vi "AppendSingle.vi"(6 "Only append if new?":bool=TRUE caption="Only append if new? (T)", 8 "Error to append":errorcluster, 9 "Error in":errorcluster) -> (1 "Appended errors out":errorcluster)   [LabVIEW 2017, in "GPError.lvlib"]
doc: "Appends <B>Error to append</B> to <B>Error in</B>.\n\nAppending errors preserves the contents of the two error clusters opposed to merging errors (with the built-in 'Merge Errors' function) which only keeps the highest priority error and scraps the rest. Appending errors maintains all error information inside the Source string of a single error cluster. Built-in, overridden and custom errors are supported.\n\nUse the SplitAppended function to split an appended error cluster into an array of individual error clusters.\n\nOnly errors and warnings are appended, any 'No error' is skipped.\n\nThe optional <B>Only append if new?</B> will, if set to True (which is the default setting), make this VI test if <B>Error to append</B> is already present in <B>Error in</B>. If that is the case (possibly as an earlier appended error) then no new append will occur. This feature is valuable if you append errors in a loop and risk encountering the same error over and over again, but you don't want to keep piling up all new copies of the same error. Set <B>Only append if new?</B> to False to append unconditionally.\n\nThis function considers two errors equal only if their code, status, source and description fields are all identical. Two errors that differ only in timestamp are considered equal as well however, the one already present in <B>Error in</B> staying put.\n\nThis VI might change the order of the appended errors, as it will always seek to move at least one error in front of any warnings in the appended error collection. This is to avoid any of the built-in LabVIEW functions wrongfully overwriting an appended error with its own error, which it will if a warning is the top-most value in the appended error collection.\n\nThis VI is reentrant.\n\nSteen Schmidt\nGPower\n18/7 2013"
uses:
  GPError.lvlib
  <vilib>/Utility/error.llb/DialogType.ctl
panel:
  # "Copyright © 2013\nSteen Schmidt, GPower\nSee enclosed license file for terms and conditions"
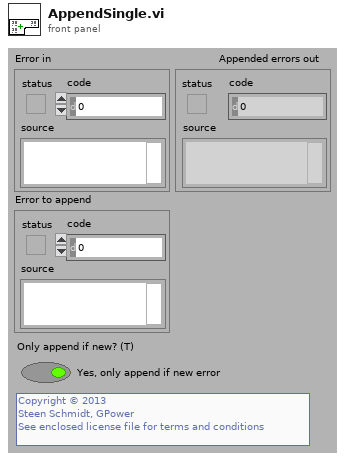
[diagram p1: front panel]
types:
  T1 = typedef "DialogType.ctl" = u16
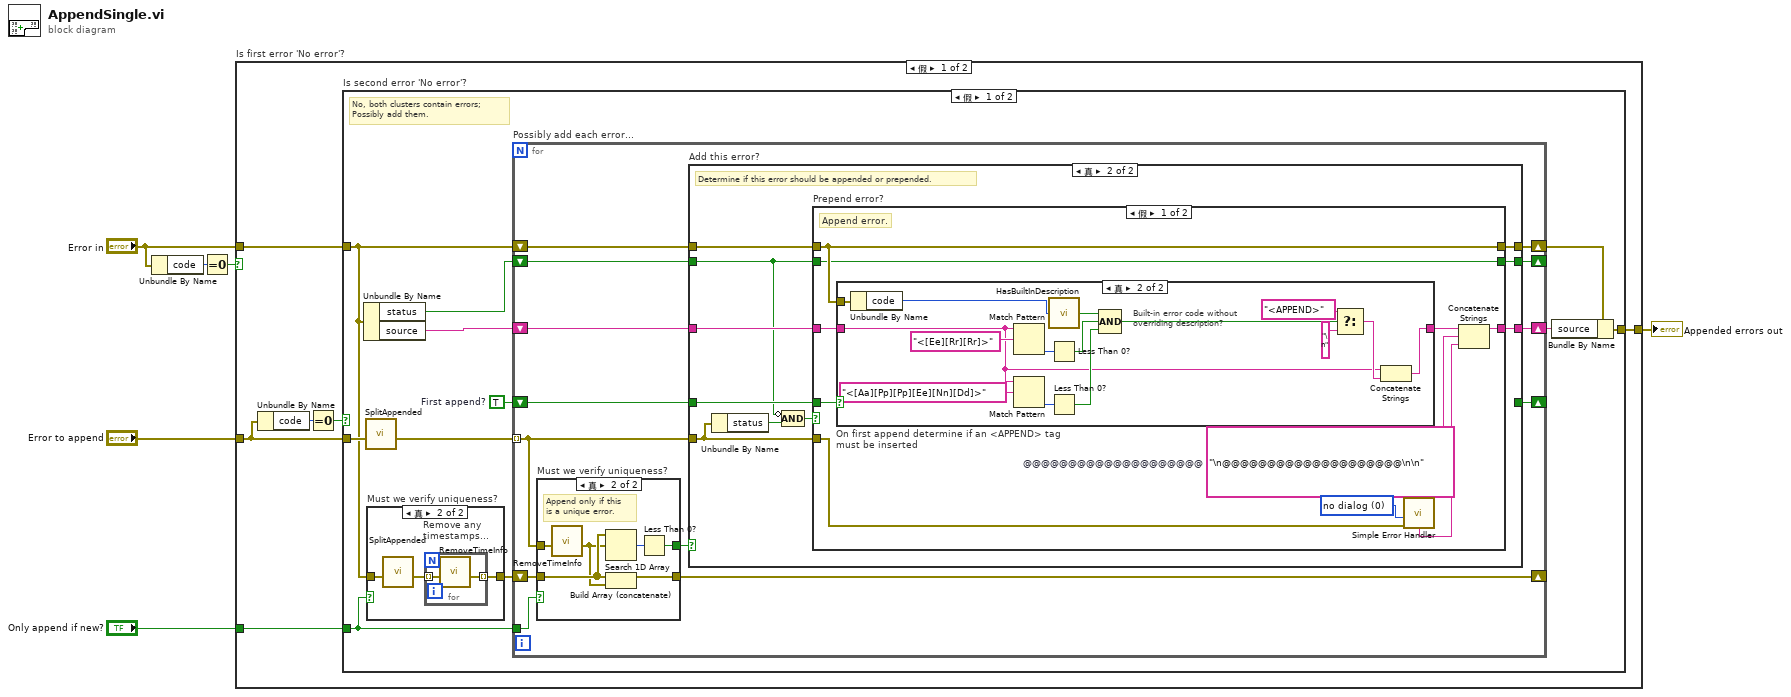
[diagram p0: block diagram]
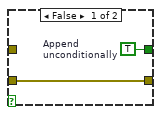
[diagram p3: hidden frame]
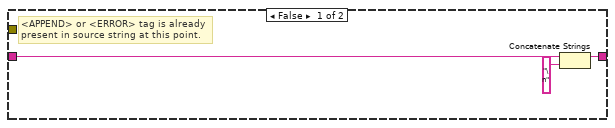
[diagram p5: hidden frame]
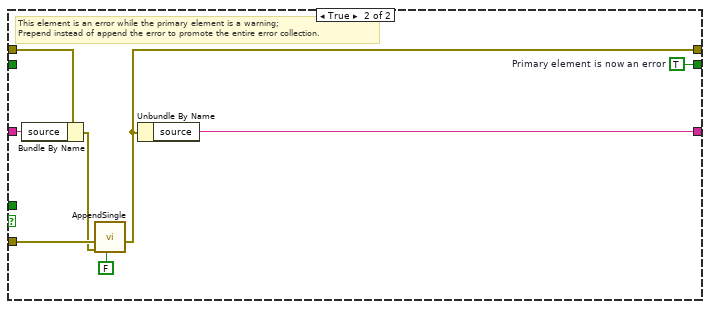
[diagram p6: hidden frame]
diagram:
  n1 = Unbundle By Name("Error in") -> ("code"=w3:i32)
  n2 = Equal To 0?(x=w3) -> (x = 0?=w1:bool)
  n3 = case "Is first error 'No error'?" shown="假" w1 {
    tunnel: [w12 w101] -> w6
    tunnel: "Error in" -> [w11 _]
    tunnel: "Error to append" -> [w8 w101]
    tunnel: "Only append if new?" -> [w10 _]
    frame False {
      n4 = Unbundle By Name(w8) -> ("code"=w9:i32)
      n5 = Equal To 0?(x=w9) -> (x = 0?=w7:bool)
      n6 = case "Is second error 'No error'?" shown="假" w7 {
        tunnel: [w19 w100] -> w12
        tunnel: w11 -> [w15 w100]
        tunnel: w8 -> [w23 _]
        tunnel: w10 -> [w21 _]
        frame False {
          w16 = TRUE  # First append?
          # "No, both clusters contain errors;\nPossibly add them."
          n7 = Unbundle By Name(w15) -> ("status"=w13:bool, "source"=w18:string)
          n8 = call "SplitAppended.vi"("Appended errors in"=w23) -> ("Errors out"=w22:errorcluster[])  [unwired: 10 in]
          n9 = case "Must we verify uniqueness?" shown="真" w21 {
            tunnel: w15 -> [_ w26]
            tunnel: [_ w24] -> w20
            frame False {
            }
            frame True {
              n10 = call "SplitAppended.vi"("Appended errors in"=w26) -> ("Errors out"=w25:errorcluster[])  [unwired: 10 in]
              n11 = for "Remove any\ntimestamps..." {
                tunnel: w25 -> [w28] mode=indexing
                tunnel: [w27] -> w24 mode=indexing
                n12 = call "RemoveTimeInfo.vi"("Error in"=w28) -> ("Error out"=w27:errorcluster)  [unwired: 9 in, 1 out]
              }
            }
          }
          n13 = for "Possibly add each error..." {
            tunnel: w22 -> [w38] mode=indexing
            shift-right: [w41] -> w17
            shift-left: w18 -> [w40]
            tunnel: w21 -> [w39]
            shift-right: [w34] -> _
            shift-left: w16 -> [w35]
            shift-right: [w33] -> _
            shift-left: w20 -> [w37]
            shift-right: [w29] -> _
            shift-left: w13 -> [w32]
            shift-right: [w30] -> w14
            shift-left: w15 -> [w31]
            n14 = case "Must we verify uniqueness?" shown="真" w39 {
              tunnel: w38 -> [_ w49]
              tunnel: w37 -> [w42 w46]
              tunnel: [w43 w47] -> w36
              tunnel: [w42 w44] -> w33
              frame False {
                w43 = TRUE  # Append unconditionally
              }
              frame True {
                # "Append only if this\nis a unique error."
                n15 = call "RemoveTimeInfo.vi"("Error in"=w49) -> ("Error out"=w45:errorcluster)  [unwired: 9 in, 1 out]
                n16 = Search 1D Array(1D array=w46, element=w45) -> (index of element=w48:i32)  [unwired: 1 in]
                n17 = Build Array (concatenate)(w46, w45) -> (w44:errorcluster[])
                n18 = Less Than 0?(x=w48) -> (x < 0?=w47:bool)
              }
            }
            n19 = case "Add this error?" shown="真" w36 {
              tunnel: [w53 w61] -> w41
              tunnel: w40 -> [w53 w63]
              tunnel: w38 -> [_ w60]
              tunnel: w35 -> [w52 w62]
              tunnel: [w52 _] -> w34
              tunnel: w32 -> [w50 w54]
              tunnel: w31 -> [w51 w57]
              tunnel: [w51 w56] -> w30
              tunnel: [w50 w55] -> w29
              frame False {
                # "Duplicate error;\nSkip it."
              }
              frame True {
                # "Determine if this error should be appended or prepended."
                n20 = Unbundle By Name(w60) -> ("status"=w59:bool)
                n21 = Compound Arithmetic op=AND(invert w54, w59) -> (w58:bool)
                n22 = case "Prepend error?" shown="假" w58 {
                  tunnel: w63 -> [w73 w98]
                  tunnel: w62 -> [w72 _]
                  tunnel: [w70 w93] -> w61
                  tunnel: w60 -> [w68 w99]
                  tunnel: w57 -> [w65 w95]
                  tunnel: [w65 w94] -> w56
                  tunnel: [w64 w92] -> w55
                  tunnel: w54 -> [w64 _]
                  frame False {
                    w69 = T1 0 items=["no dialog", "OK message", "continue or stop message", "OK message + warnings", "continue/stop + warnings"] ("type of dialog (OK msg:1)")
                    w67 = "\n@@@@@@@@@@@@@@@@@@@@\n\n"  # @@@@@@@@@@@@@@@@@@@@
                    # "Append error."
                    n23 = case "On first append determine if an <APPEND> tag must be inserted" shown="真" w72 {
                      tunnel: w65 -> [_ w78]
                      tunnel: w73 -> [w76 w80]
                      tunnel: [w75 w79] -> w71
                      frame False {
                        # "<APPEND> or <ERROR> tag is already\npresent in source string at this point."
                        n24 = Concatenate Strings(w76, "\n") -> (w75:string)
                      }
                      frame True {
                        # "Built-in error code without\noverriding description?"
                        n25 = Unbundle By Name(w78) -> ("code"=w77:i32)
                        n26 = Match Pattern(string=w80, regular expression="<[Ee][Rr][Rr]>") -> (offset past match=w90:i32)  [unwired: 1 in, 3 out]
                        n27 = Match Pattern(string=w80, regular expression="<[Aa][Pp][Pp][Ee][Nn][Dd]>") -> (offset past match=w83:i32)  [unwired: 1 in, 3 out]
                        n28 = call "HasBuiltInDescription.vi"("Error/warning code"=w77) -> ("Has built-in description?"=w89:bool)  [unwired: 4 in]
                        n29 = Less Than 0?(x=w90) -> (x < 0?=w88:bool)
                        n30 = Less Than 0?(x=w83) -> (x < 0?=w81:bool)
                        n31 = Compound Arithmetic op=AND(w89, w88, w81) -> (w87:bool)
                        n32 = Select(t="<APPEND>", s=w87, f="\n") -> (s? t:f=w85:string)
                        n33 = Concatenate Strings(w80, w85) -> (w79:string)
                      }
                    }
                    n34 = call <vilib>:"Simple Error Handler.vi"("type of dialog (OK msg:1)"=w69, "error in (no error)"=w68) -> ("message"=w66:string)  [unwired: 3 in, 4 out]
                    n35 = Concatenate Strings(w71, w67, w66) -> (w70:string)
                  }
                  frame True {
                    w92 = TRUE  # Primary element is now an error
                    # "This element is an error while the primary element is a warning;\nPrepend instead of append the error to promote the entire error collection."
                    n36 = Bundle By Name(cluster=w95, "source"=w98) -> (w97:errorcluster)
                    n37 = call "AppendSingle.vi"("Only append if new?"=FALSE, "Error to append"=w97, "Error in"=w99) -> ("Appended errors out"=w94:errorcluster)  [unwired: 8 in]
                    n38 = Unbundle By Name(w94) -> ("source"=w93:string)
                  }
                }
              }
            }
          }
          n39 = Bundle By Name(cluster=w14, "source"=w17) -> (w19:errorcluster)
        }
        frame True {
          # "Just return first error."
        }
      }
    }
    frame True {
      # "Just return second error."
    }
  }
  "Appended errors out" <- w6
